vi "WPI_Camera HTTP Connection Respondervi.vi"(9 "CGI String":string="stream.mjpg", 10 "parameters":T1(array[cluster]), 11 "connection ID":refnum<k5>) -> ()   [LabVIEW 2018]
doc: "This VI is launched each time a new client camera connection is requested. The connection will remain open until closed by the client or because of errors with the camera. Parameters are name/lvalue pairs that have been parsed from a URL request. Supported parameters are name, fps, resolution, compression, exposure, brightness, whitebalance, sharpness, and colorlevel.\n\nThe first four parameters are filled with defaults if not provided, but the latter four are only set if provided."
uses:
  Error Cluster From Error Code.vi
  Error Ring.xnode
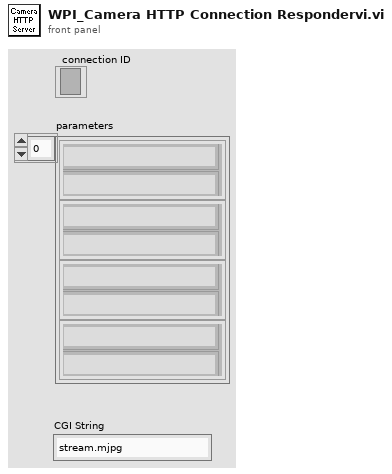
[diagram p1: front panel]
types:
  T1 = cluster{"token string":string, "token string 2":string}[]
  T2 = cluster{"White Balance":string, "Brightness":i32, "Sharpness":i32, "Saturation":i32, "Exposure":string}
  T3 = cluster{"Camera Name":string, "Size":string, "Frame Rate":i32, "Compression":i32}
  T4 = enum8{"Controller", "Module", "Language", "CANPlugin", "Accelerometer", "ADXL345", "AnalogChannel", "AnalogTrigger", "AnalogTriggerOutput", "CANJaguar", "Compressor", "Counter", "Dashboard", "DigitalInput", "DigitalOutput", "DriverStationCIO", "DriverStationEIO", "DriverStationLCD", "Encoder", "GearTooth", "Gyro", "I2C", "Framework", "Jaguar", "Joystick", "Kinect", "KinectStick", "PIDController", "Preferences", "PWM", "Relay", "RobotDrive", "SerialPort", "Servo", "Solenoid", "SPI", "Task", "Ultrasonic", "Victor", "Button", "Command", "AxisCamera", "PCVideoServer", "SmartDashboard", "Talon", "HiTechnicColorSensor", "HiTechnicAccel", "HiTechnicCompass", "SRF08", "AnalogOutput", "Victor SP", "Talon SRX", "CAN Talon SRX", "ADXL362 Accel", "ADXRS450 Gyro", "Rev SPARK", "Mindsensors SD540", "Digital Filter", "ADIS16448", "PDP", "PCM", "PigeonIMU", "Nidec Brushless", "CTRE CANifier", "CTRE Future 0", "CTRE Future 1", "CTRE Future 2", "CTRE Future 3", "CTRE Future 4", "CTRE Future 5", "CTRE Future 6", "Linear Filter", "Xbox Controller", "USB Camera", "NavX", "Pixy", "Pixy2", "ScanseSweep", "Shuffleboard", "CAN", "Digilent DMC60", "PWM Victor SPX", "Rev SPARK MAX PWM", "Rev SPARK MAX CAN", "ADIS16470"}
  T5 = cluster{"White Balance":bool, "Brightness":bool, "Sharpness":bool, "Saturation":bool, "Exposure":bool}
  T6 = cluster{"Camera Address":string, "CameraStatus":errorcluster}
  T7 = enum16{"640x480", "320x240", "160x120", "Custom"}
  T8 = typedef "IMAQ Image.ctl" = refnum<image>
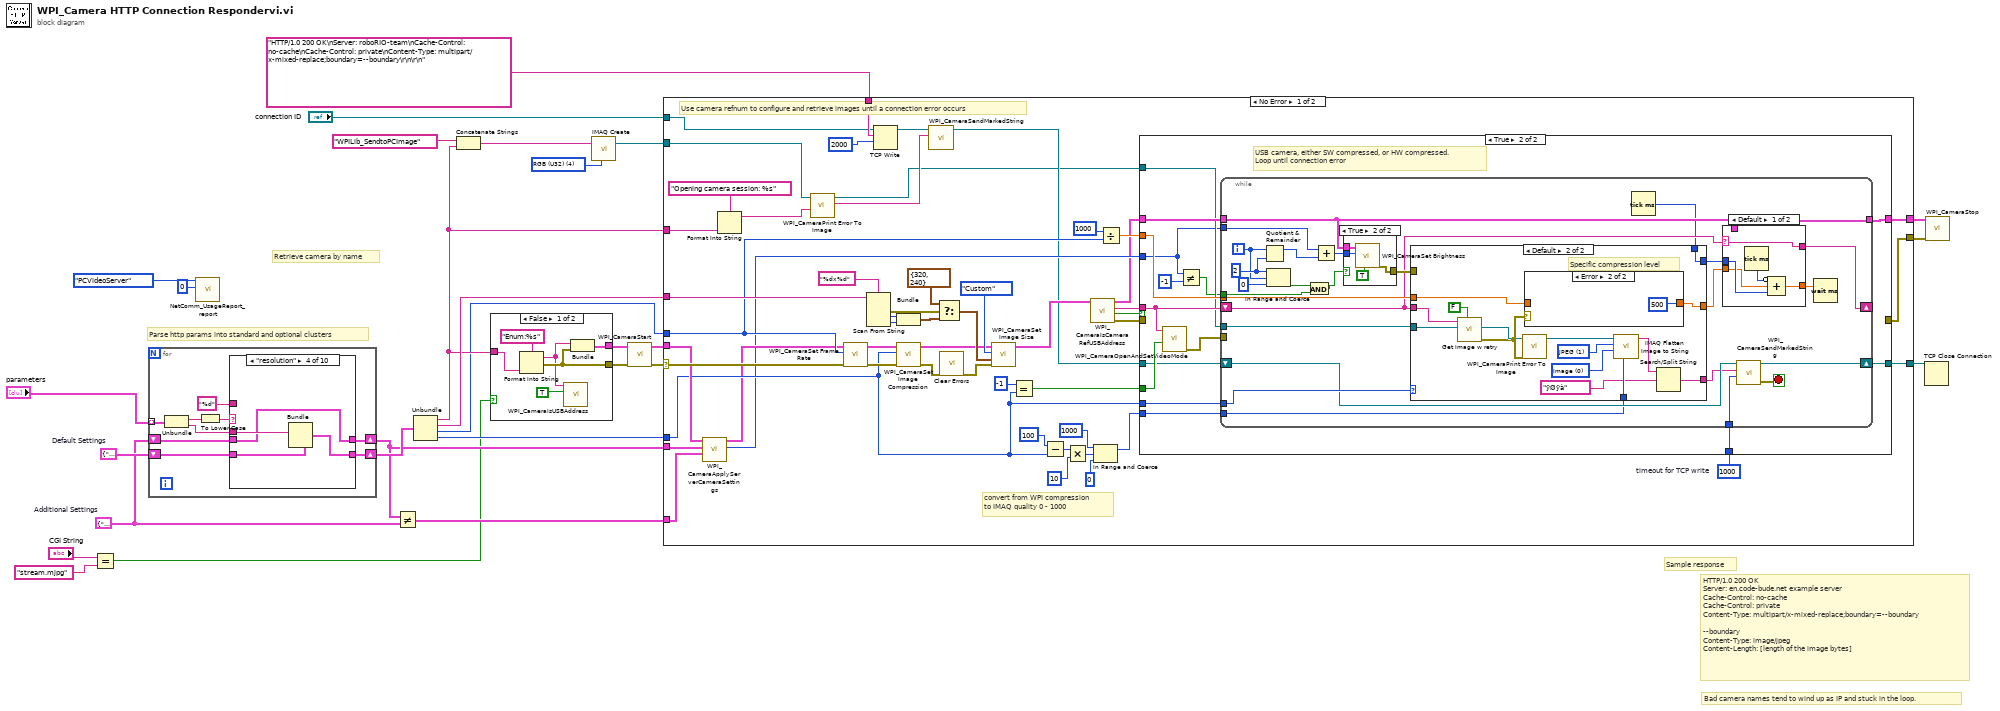
[diagram p0: block diagram]
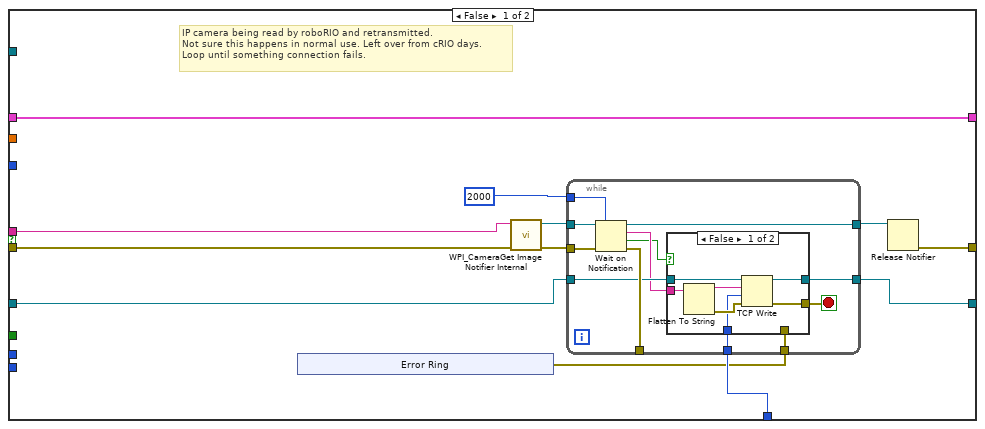
[diagram p2: hidden frame]
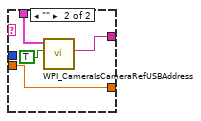
[diagram p4: hidden frame]
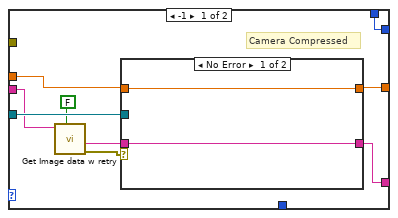
[diagram p6: hidden frame]
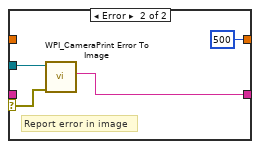
[diagram p7: hidden frame]
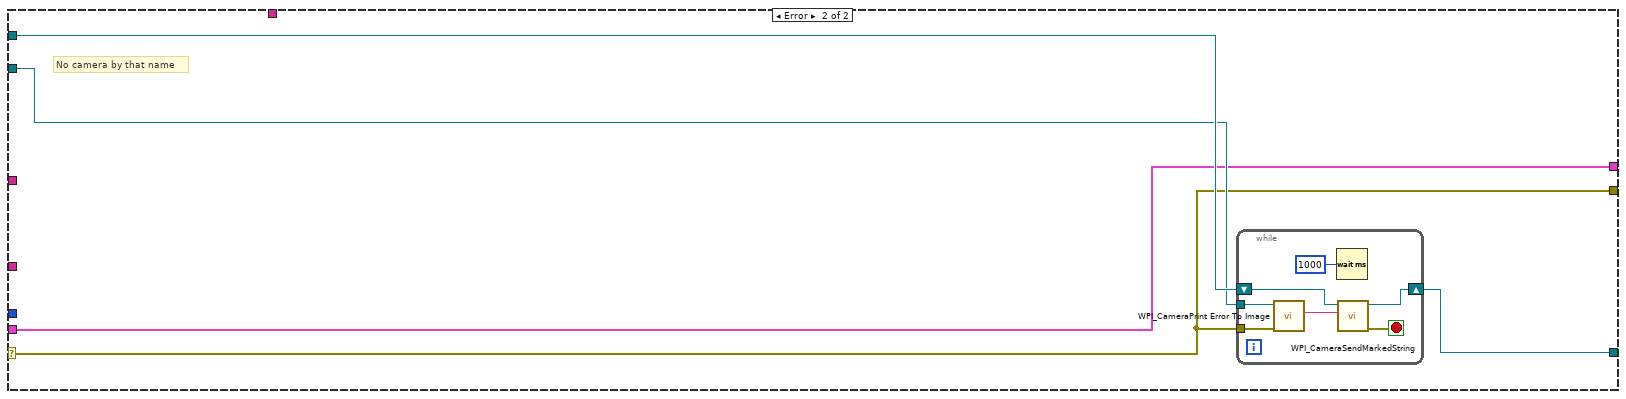
[diagram p9: hidden frame]
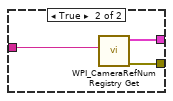
[diagram p10: hidden frame]
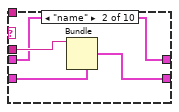
[diagram p12: hidden frame]
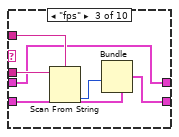
[diagram p13: hidden frame]
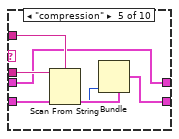
[diagram p14: hidden frame]
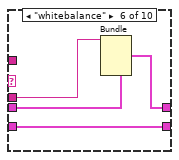
[diagram p15: hidden frame]
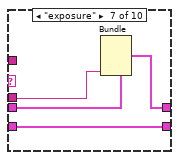
[diagram p16: hidden frame]
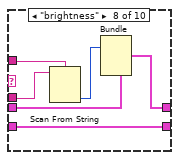
[diagram p17: hidden frame]
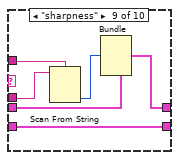
[diagram p18: hidden frame]
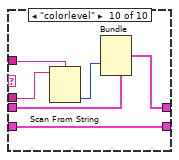
[diagram p19: hidden frame]
diagram:
  w14 = u32 4 items=["Grayscale (U8)", "Grayscale (I16)", "Grayscale (SGL)", "Complex (CSG)", "RGB (U32)", "HSL (U32)", "RGB (U64)", "Grayscale (U16)"] ("Image Type")
  w20 = T2 {"White Balance"="", "Brightness"=-1, "Sharpness"=-1, "Saturation"=-1, "Exposure"=""}  # Additional Settings
  w25 = T3 {"Camera Name"="Camera", "Size"="320x240", "Frame Rate"=15, "Compression"=30}  # Default Settings
  # "Sample response"
  # "HTTP/1.0 200 OK\nServer: en.code-bude.net example server\nCache-Control: no-cache\nCache-Control: private\nContent-Type: multipart/x-mixed-replace;boundary=--boundary\n \n--boundary\nContent-Type: image/jpeg\nContent-Length: [length of the image bytes]"
  # "Retrieve camera by name"
  # "Parse http params into standard and optional clusters"
  # "Bad camera names tend to wind up as IP and stuck in the loop."
  n1 = Equal?(x="CGI String", y="stream.mjpg" ("CGI String")) -> (x = y?=w7:bool)
  n2 = for {
    tunnel: "parameters" -> [w37] mode=indexing
    shift-right: [w32] -> w23
    shift-left: w25 -> [w34]
    shift-right: [w29] -> w18
    shift-left: w20 -> [w30]
    n3 = Unbundle(w37) -> ("token string"=w36:string, "token string 2"=w33:string)
    n4 = To Lower Case(string=w36) -> (all lower case string=w35:string)
    n5 = case shown="\"resolution\"" w35 {
      tunnel: w34 -> [w39 w43 w49 w53 w59 w63 w67 w73 w79 w85]
      tunnel: w33 -> [_ w42 w47 w51 w57 w61 w64 w69 w75 w81]
      tunnel: [w39 w41 w48 w52 w58 w63 w67 w73 w79 w85] -> w32
      tunnel: "%d" -> [_ _ w46 _ w55 _ _ w70 w76 w82]
      tunnel: w30 -> [w38 w40 w44 w50 w54 w62 w66 w72 w78 w84]
      tunnel: [w38 w40 w44 w50 w54 w60 w65 w71 w77 w83] -> w29
      frame Default {
      }
      frame "name" {
        n6 = Bundle(cluster=w43, "Camera Name"=w42) -> (w41:T3)  [unwired: 3 in]
      }
      frame "fps" {
        n7 = Scan From String(format string=w46, input string=w47) -> (output 1=w45:i32)  [unwired: 3 in, 3 out]
        n8 = Bundle(cluster=w49, "Frame Rate"=w45) -> (w48:T3)  [unwired: 3 in]
      }
      frame "resolution" {
        n9 = Bundle(cluster=w53, "Size"=w51) -> (w52:T3)  [unwired: 3 in]
      }
      frame "compression" {
        n10 = Scan From String(format string=w55, input string=w57) -> (output 1=w56:i32)  [unwired: 3 in, 3 out]
        n11 = Bundle(cluster=w59, "Compression"=w56) -> (w58:T3)  [unwired: 3 in]
      }
      frame "whitebalance" {
        n12 = Bundle(cluster=w62, "White Balance"=w61) -> (w60:T2)  [unwired: 4 in]
      }
      frame "exposure" {
        n13 = Bundle(cluster=w66, "Exposure"=w64) -> (w65:T2)  [unwired: 4 in]
      }
      frame "brightness" {
        n14 = Scan From String(format string=w70, input string=w69) -> (output 1=w68:i32)  [unwired: 3 in, 3 out]
        n15 = Bundle(cluster=w72, "Brightness"=w68) -> (w71:T2)  [unwired: 4 in]
      }
      frame "sharpness" {
        n16 = Scan From String(format string=w76, input string=w75) -> (output 1=w74:i32)  [unwired: 3 in, 3 out]
        n17 = Bundle(cluster=w78, "Sharpness"=w74) -> (w77:T2)  [unwired: 4 in]
      }
      frame "colorlevel" {
        n18 = Scan From String(format string=w82, input string=w81) -> (output 1=w80:i32)  [unwired: 3 in, 3 out]
        n19 = Bundle(cluster=w84, "Saturation"=w80) -> (w83:T2)  [unwired: 4 in]
      }
    }
  }
  n20 = call "NetComm_UsageReport_report.vi"("Instance Number"=u8 0, "Resource Type"=T4."PCVideoServer") -> ()  [unwired: 10 in]
  n21 = Not Equal?(x=w18, y=w20) -> (x != y?=w19:T5)
  n22 = Unbundle(w23) -> ("Camera Name"=w12:string, "Size"=w24:string, "Frame Rate"=w8:i32, "Compression"=w17:i32)
  n23 = Concatenate Strings("WPILib_SendtoPCImage", w12) -> (w13:string)
  n24 = case shown="False" w7 {
    tunnel: [w89 w94] -> w3
    tunnel: [w88 w93] -> w5
    tunnel: w12 -> [w91 w92]
    frame False {
      n25 = Format Into String(format string="Enum:%s" ("Camera Address"), w91) -> (resulting string=w87:string, error out=w88:errorcluster)  [unwired: 2 in]
      n26 = call "WPI_CameraIsUSBAddress.vi"("Enumerate?"=TRUE, "Camera Address In"=w87) -> ()  [unwired: 7 in, 3 out]
      n27 = Bundle(w87, "error IO"=w88) -> (w89:cluster{string, "error IO":errorcluster})  [unwired: 1 in]
    }
    frame True {
      n28 = call "WPI_CameraRefNum Registry Get.vi"("refnum name"=w92) -> ("error out"=w93:errorcluster, "CameraDevRef"=w94:T6)  [unwired: 9 in]
    }
  }
  n29 = call "IMAQ Create"("Image Name"=w13, "Image Type"=w14) -> ("New Image"=w15:refnum<image>)  [unwired: 3 in, 1 out]
  n30 = call "WPI_CameraStart.vi"("error in (no error)"=w5, "CameraDevRef"=w3) -> ("error out"=w6:errorcluster, "CameraDevRef"=w4:T6)  [unwired: 8 out]
  n31 = case shown="No Error" w6 {
    selector: w6 -> [w124 w271]
    tunnel: [w147 w274] -> w28
    tunnel: w4 -> [w116 w272]
    tunnel: w24 -> [w135 _]
    tunnel: w19 -> [w126 _]
    tunnel: w18 -> [w125 _]
    tunnel: w17 -> [w115 _]
    tunnel: w8 -> [w123 _]
    tunnel: "connection ID" -> [w103 w275]
    tunnel: w15 -> [w108 w273]
    tunnel: w12 -> [w110 _]
    tunnel: "HTTP/1.0 200 OK\nServer: roboRIO-team\nCache-Control: no-cache\nCache-Control: private\nContent-Type: multipart/x-mixed-replace;boundary=--boundary\r\n\r\n" ("regular expression") -> [w104 _]
    tunnel: [w101 w271] -> w2
    tunnel: [w100 w272] -> w1
    frame No Error {
      w95 = 1000  # timeout for TCP write
      # "Use camera refnum to configure and retrieve images until a connection error occurs"
      # "convert from WPI compression\nto IMAQ quality 0 - 1000"
      n32 = call "WPI_CameraApplyServerCameraSettings.vi"("Unique"=w126, "Additional Settings"=w125, "CameraDevRef"=w116) -> ("Brightness"=w113:i32, "CameraDevRef Out"=w114:T6)  [unwired: 7 in]
      n33 = Format Into String(format string="Opening camera session: %s", w110) -> (resulting string=w106:string)  [unwired: 2 in, 1 out]
      n34 = call "WPI_CameraPrint Error To Image.vi"("String"=w106, "Image"=w108) -> ("flattened error string"=w112:string, "Image out"=w107:T8)  [unwired: 8 in]
      n35 = call "WPI_CameraSet Frame Rate.vi"("error in (no error)"=w124, "Frame Rate (fps)"=w123, "CameraDevRef"=w114) -> ("error out"=w120:errorcluster, "CameraDevRef Out"=w122:T6)  [unwired: 7 in]
      n36 = Scan From String(format string="%dx%d", input string=w135) -> (error out=w130:errorcluster, output 1=w133:i32, output 2=w132:i32)  [unwired: 4 in, 2 out]
      n37 = TCP Write(connection ID=w103, data in=w104, 9:2000) -> (connection ID out=w102:refnum<k5>)  [unwired: 1 in, 2 out]
      n38 = Bundle(w133, w132) -> (w129:cluster{i32, i32})  [unwired: 1 in]
      n39 = call "WPI_CameraSet Image Compression.vi"("error in (no error)"=w120, "Compression"=w115, "CameraDevRef"=w122) -> ("error out"=w119:errorcluster, "CameraDevRef Out"=w121:T6)  [unwired: 7 in]
      n40 = call "WPI_CameraSendMarkedString.vi"("Data String"=w112, "TCP Network Connection in"=w102) -> ("TCP Network Connection out"=w111:refnum<k5>)  [unwired: 8 in, 1 out]
      n41 = Select(t=cluster{i32, i32} {320, 240} ("s? t:f"), s=w130, f=w129) -> (s? t:f=w128:cluster{i32, i32})
      n42 = call "Clear Errors.vi"("error in (no error)"=w119) -> ("error out"=w118:errorcluster)  [unwired: 5 in, 1 out]
      n43 = call "WPI_CameraSet Image Size.vi"("error in (no error)"=w118, "Size W,H (pix)"=w128, "Image Size"=T7."Custom", "CameraDevRef"=w121) -> ("CameraDevRef Out"=w117:T6)  [unwired: 6 in, 1 out]
      n44 = Equal?(x=-1, y=w115) -> (x = y?=w136:bool)
      n45 = Subtract(x=100, y=w115) -> (x-y=w140:i32)
      n46 = Multiply(x=w140, y=10) -> (x*y=w142:i32)
      n47 = call "WPI_CameraIsCameraRefUSBAddress.vi"("CameraDevRef"=w117) -> ("error out"=w96:errorcluster, "USB?"=w98:bool, "Camera Address Out"=w99:string, "CameraDevRef out"=w97:T6)  [unwired: 7 in]
      n48 = In Range and Coerce(upper limit=1000, x=w142, lower limit=0) -> (coerced(x)=w138:i32)  [unwired: 1 out]
      n49 = Divide(x=u16 1000 ("port"), y=w123) -> (x/y=w145:dbl)
      n50 = case shown="True" w98 {
        tunnel: w111 -> [w159 w188]
        tunnel: [w158 w199] -> w147
        tunnel: w96 -> [w157 _]
        tunnel: w99 -> [w155 w195]
        tunnel: [w149 w197] -> w100
        tunnel: w97 -> [w149 w198]
        tunnel: [w153 _] -> w101
        tunnel: w138 -> [_ w192]
        tunnel: w145 -> [_ w190]
        tunnel: w115 -> [_ w196]
        tunnel: w136 -> [_ w194]
        tunnel: w95 -> [w151 w193]
        tunnel: w113 -> [_ w187]
        tunnel: w107 -> [_ w189]
        frame False {
          # "IP camera being read by roboRIO and retransmitted.\nNot sure this happens in normal use. Left over from cRIO days.\nLoop until something connection fails."
          n51 = xnode "Error Ring"() -> ("error out"=w148:errorcluster)
          n52 = call "WPI_CameraGet Image Notifier Internal.vi"("error in (no error)"=w157, "Camera Address"=w155) -> ("error out"=w156:errorcluster, "Image Notifier"=w154:refnum<notifier>)  [unwired: 8 out]
          n53 = while {
            tunnel: w156 -> [w175]
            tunnel: w159 -> [w170]
            tunnel: [w173] -> _
            tunnel: [w169] -> w158
            tunnel: w154 -> [w174]
            tunnel: [w172] -> w152
            tunnel: w151 -> [w171]
            tunnel: w148 -> [w166]
            tunnel: 2000 ("Timeout in ms (-1)") -> [w165]
            stop <- w164 stop-if-true
            n54 = Wait on Notification(notifier=w174, timeout in ms (-1)=w165, error in (no error)=w175) -> (notifier out=w172:refnum<notifier>, notification=w168:string, timed out?=w167:bool, error out=w173:errorcluster)  [unwired: 1 out]
            n55 = case shown="False" w167 {
              tunnel: [w180 w183] -> w164
              tunnel: w171 -> [w179 _]
              tunnel: w170 -> [w178 w184]
              tunnel: [w176 w184] -> w169
              tunnel: w168 -> [w177 _]
              tunnel: w166 -> [_ w183]
              frame False {
                n56 = Flatten To String(anything=w177) -> (data string=w182:string, error out=w181:errorcluster)  [unwired: 1 in, 3 out]
                n57 = TCP Write(connection ID=w178, data in=w182, error in (no error)=w181, 9:w179) -> (connection ID out=w176:refnum<k5>, error out=w180:errorcluster)  [unwired: 1 out]
              }
              frame True {
              }
            }
          }
          n58 = Release Notifier(notifier=w152) -> (error out=w153:errorcluster)  [unwired: 1 in, 3 out]
        }
        frame True {
          # "USB camera, either SW compressed, or HW compressed.\nLoop until connection error"
          n59 = call "WPI_CameraOpenAndSetVideoMode.vi"("USB JPEG"=w194, "Camera Address"=w195) -> ("error out"=w191:errorcluster)  [unwired: 9 in]
          n60 = Not Equal?(x=w187, y=-1 ("port")) -> (x != y?=w185:bool)
          n61 = while {
            shift-right: [w219] -> w199
            shift-left: w188 -> [w224]
            tunnel: [w213] -> w197
            tunnel: w198 -> [w213]
            tunnel: w196 -> [w225]
            tunnel: w193 -> [w223]
            tunnel: w192 -> [w222]
            tunnel: w191 -> [_]
            tunnel: w190 -> [w218]
            tunnel: w187 -> [w204]
            shift-right: [w214] -> _
            shift-left: w195 -> [w212]
            tunnel: w189 -> [w211]
            tunnel: w185 -> [w201]
            i -> [w200]
            stop <- w220 stop-if-true
            w205 = u16 2 ("port")
            n62 = Quotient & Remainder(x=w200, y=w205) -> (x-y*floor(x/y)=w216:i32)  [unwired: 1 out]
            n63 = In Range and Coerce(upper limit=w205, x=w200, lower limit=u16 0 ("port")) -> (In Range?=w203:bool)  [unwired: 1 out]
            n64 = And(x=w203, y=w201) -> (x .and. y?=w202:bool)
            n65 = Add(x=w204, y=w216) -> (x+y=w215:i32)
            n66 = case shown="True" w202 {
              tunnel: w213 -> [_ w238]
              tunnel: [_ w237] -> w217
              tunnel: w215 -> [_ w236]
              frame False {
              }
              frame True {
                n67 = call "WPI_CameraSet Brightness.vi"("Force"=TRUE, "Brightness"=w236, "CameraDevRef"=w238) -> ("error out"=w237:errorcluster)  [unwired: 7 in, 1 out]
              }
            }
            n68 = Tick Count (ms)() -> (millisecond timer value=w208:u32)
            n69 = case shown="Default" w225 {
              tunnel: [w247 w265] -> w221
              tunnel: w212 -> [w240 w258]
              tunnel: w211 -> [w246 w257]
              tunnel: w222 -> [_ w266]
              tunnel: w218 -> [w245 w261]
              tunnel: [w244 w260] -> w210
              tunnel: w217 -> [_ _]
              tunnel: [w243 w259] -> w209
              tunnel: w208 -> [w243 w259]
              frame -1 {
                # "Camera Compressed"
                n70 = call "Get Image data w retry.vi"("Wait"=FALSE ("DB"), "Session In"=w240) -> ("error out"=w241:errorcluster, "Image Data String"=w242:string)  [unwired: 6 in, 2 out]
                n71 = case shown="No Error" w241 {
                  selector: w241 -> [_ w253]
                  tunnel: [w249 w250] -> w247
                  tunnel: w242 -> [w249 _]
                  tunnel: w246 -> [_ w252]
                  tunnel: w245 -> [w248 _]
                  tunnel: [w248 u16 500 ("port")] -> w244
                  frame No Error {
                  }
                  frame Error {
                    # "Report error in image"
                    n72 = call "WPI_CameraPrint Error To Image.vi"("error in (no error)"=w253, "Image"=w252) -> ("flattened error string"=w250:string)  [unwired: 8 in, 1 out]
                  }
                }
              }
              frame Default {
                w267 = 0 items=["Image", "Image and Vision Info", "Reference to Image"] ("Type of Flatten (Image and Vision Info)")
                w268 = 1 items=["None", "JPEG", "PACKED BINARY"] ("Compression (None)")
                # "Specific compression level"
                n73 = call "Get Image w retry.vi"("Wait"=FALSE, "Image In"=w257, "Session In"=w258) -> ("error out"=w255:errorcluster, "Image Out"=w256:refnum<image>)  [unwired: 6 in, 1 out]
                n74 = call "WPI_CameraPrint Error To Image.vi"("error in (no error)"=w255, "Image"=w256) -> ("Image out"=w263:T8)  [unwired: 8 in, 1 out]
                n75 = case shown="Error" w255 {
                  tunnel: w261 -> [w269 _]
                  tunnel: [w269 500] -> w260
                  frame No Error {
                  }
                  frame Error {
                  }
                }
                n76 = call "IMAQ Flatten Image to String"("Quality (750)"=w266, "Type of Flatten (Image and Vision Info)"=w267, "Compression (None)"=w268, "Image"=w263) -> ("Data String"=w264:string)  [unwired: 6 in, 1 out]
                n77 = Search/Split String(string=w264, search string/char (-)="ÿØÿà" ("format string")) -> (match + rest of string=w265:string)  [unwired: 1 in, 2 out]
              }
            }
            n78 = case shown="Default" w212 {
              selector: w212 -> [w230 _]
              tunnel: w213 -> [_ w234]
              tunnel: [w230 w233] -> w214
              tunnel: w210 -> [w227 w231]
              tunnel: w209 -> [w229 _]
              tunnel: [w228 w231] -> w207
              frame Default {
                n79 = Tick Count (ms)() -> (millisecond timer value=w226:u32)
                n80 = Compound Arithmetic op=ADD(invert w226, w227, w229) -> (w228:dbl)
              }
              frame "" {
                n81 = call "WPI_CameraIsCameraRefUSBAddress.vi"("Enumerate"=TRUE ("Enumerate?"), "CameraDevRef"=w234) -> ("Camera Address Out"=w233:string)  [unwired: 6 in, 3 out]
              }
            }
            n82 = call "WPI_CameraSendMarkedString.vi"("timeout for TCP write"=w223, "Data String"=w221, "TCP Network Connection in"=w224) -> ("error out"=w220:errorcluster, "TCP Network Connection out"=w219:refnum<k5>)  [unwired: 7 in]
            n83 = Wait (ms)(milliseconds to wait=w207) -> ()  [unwired: 1 out]
          }
        }
      }
    }
    frame Error {
      # "No camera by that name"
      n84 = while {
        shift-right: [w276] -> w274
        shift-left: w275 -> [w277]
        tunnel: w271 -> [w282]
        tunnel: w273 -> [w281]
        stop <- w279 stop-if-true
        n85 = call "WPI_CameraPrint Error To Image.vi"("error in (no error)"=w282, "Image"=w281) -> ("flattened error string"=w278:string)  [unwired: 8 in, 1 out]
        n86 = Wait (ms)(milliseconds to wait=u32 1000) -> ()  [unwired: 1 out]
        n87 = call "WPI_CameraSendMarkedString.vi"("Data String"=w278, "TCP Network Connection in"=w277) -> ("error out"=w279:errorcluster, "TCP Network Connection out"=w276:refnum<k5>)  [unwired: 8 in]
      }
    }
  }
  n88 = TCP Close Connection(connection ID=w28) -> ()  [unwired: 1 in, 3 out]
  n89 = call "WPI_CameraStop.vi"("error in (no error)"=w2, "CameraDevRef"=w1) -> ()  [unwired: 10 out]
